vi "test Get Set EST CD.vi"(8 "error in (no error)":errorcluster, 11 "TestCase in":refnum<class "Scripting API Test Case.lvclass">) -> (0 "error out":errorcluster, 3 "TestCase out":refnum<class "Scripting API Test Case.lvclass">)   [LabVIEW 2020, in "Scripting API Test Case.lvclass"]
uses:
  Scripting API Test Case.lvclass
  Scripting API/Custom Device/Engine Simulation Toolkit Custom Device Settings.ctl
  Scripting API Test Case.lvclass/Scripting API Test Case.ctl
  <vilib>/addons/_JKI Toolkits/VI Tester/TestCase.llb/TestCase.lvclass
  Scripting API/Engine Simulation Toolkit Scripting API.lvlib
  C:/Program Files (x86)/National Instruments/LabVIEW 2020/vi.lib/addons/_JKI Toolkits/VI Tester/TestCase.llb/TestCase.lvclass
panel:
  in  "Save?":bool
  out "Output Filename":string
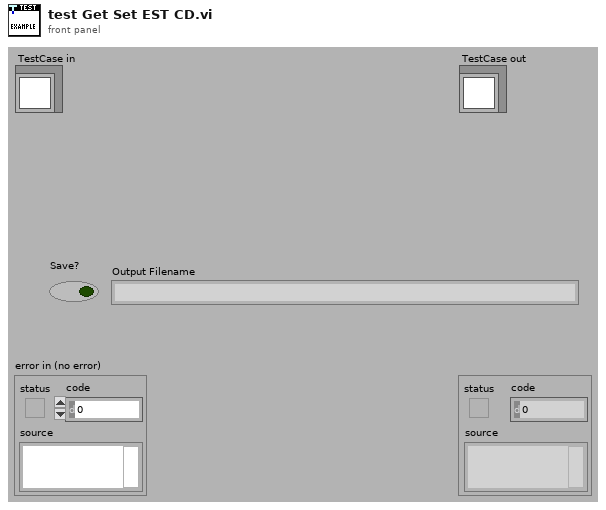
[diagram p1: front panel]
types:
  T1 = typedef "Engine Simulation Toolkit Scripting API.lvlib/Engine Simulation Toolkit Custom Device Settings.ctl" = cluster{"Name":string, "Execution priority":enum16{"Low", "Medium", "High"}, "Rate decimation":i32, "CPU":i32}
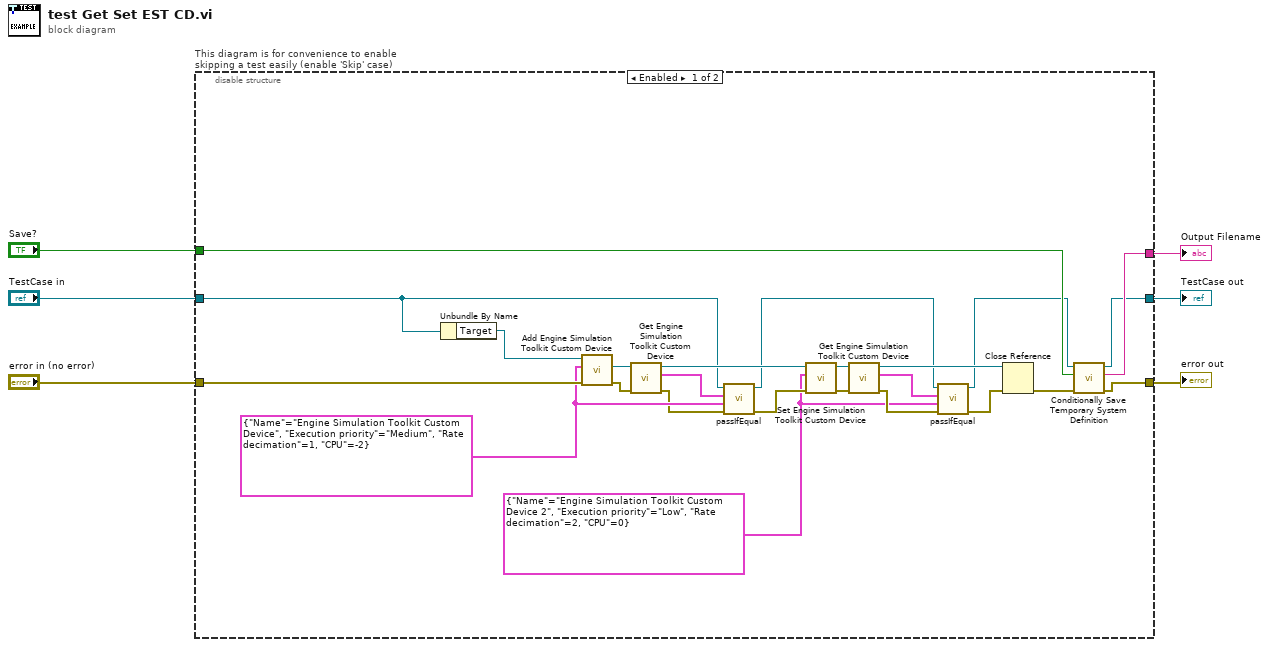
[diagram p0: block diagram]
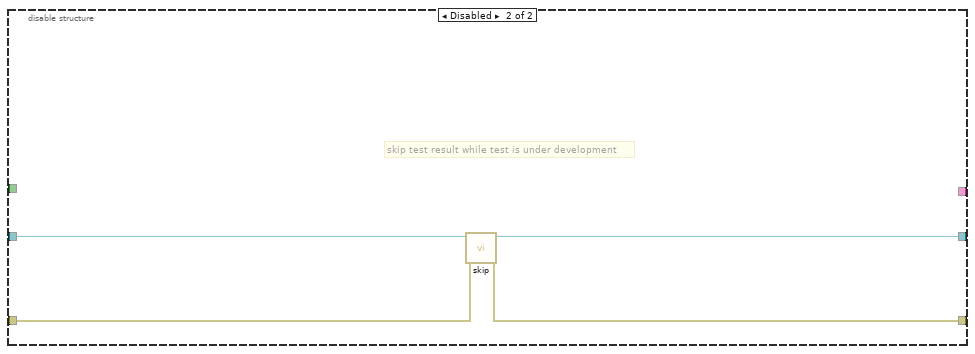
[diagram p2: hidden frame]
diagram:
  n1 = disable-structure "This diagram is for convenience to enable skipping a test easily (enable 'Skip' case)" shown="Enabled" {
    disable-tunnel: "TestCase in" -> [w10 w34]
    disable-tunnel: [w7 w32] -> w3
    disable-tunnel: [w29 w33] -> w5
    disable-tunnel: "error in (no error)" -> [w30 w31]
    disable-tunnel: [w28 _] -> w2
    disable-tunnel: "Save?" -> [w27 _]
    frame Enabled {
      w11 = T1 {"Name"="Engine Simulation Toolkit Custom Device 2", "Execution priority"=enum."Low", "Rate decimation"=2, "CPU"=0} ("Engine Simulation Toolkit Custom Device Settings")
      w20 = T1 {"Name"="Engine Simulation Toolkit Custom Device", "Execution priority"=enum."Medium", "Rate decimation"=1, "CPU"=-2} ("Engine Simulation Toolkit Custom Device Settings")
      n2 = Unbundle By Name(w10) -> ("Target"=w9:refnum<k24>)
      n3 = call "Add Engine Simulation Toolkit Custom Device.vi"("error in (no error)"=w30, "Settings"=w20, "Target in"=w9) -> ("error out"=w23:errorcluster, "EST Custom Device"=w22:refnum<k24>)  [unwired: 6 in, 1 out]
      n4 = call "Get Engine Simulation Toolkit Custom Device.vi"("error in (no error)"=w23, "EST Custom Device in"=w22) -> ("error out"=w16:errorcluster, "Settings"=w21:T1, "EST Custom Device out"=w24:refnum<k24>)  [unwired: 7 in]
      n5 = call-dynamic "passIfEqual.vi"("error in (no error)"=w16, "y"=w20, "x"=w21, "TestCase in"=w10) -> ("error out"=w17:errorcluster, "TestCase out"=w13:refnum<class "Scripting API Test Case.lvclass">)  [unwired: 6 in]
      n6 = call "Set Engine Simulation Toolkit Custom Device.vi"("error in (no error)"=w17, "Settings"=w11, "EST Custom Device in"=w24) -> ("error out"=w26:errorcluster, "EST Custom Device out"=w25:refnum<k24>)  [unwired: 7 in]
      n7 = call "Get Engine Simulation Toolkit Custom Device.vi"("error in (no error)"=w26, "EST Custom Device in"=w25) -> ("error out"=w15:errorcluster, "Settings"=w12:T1, "EST Custom Device out"=w18:refnum<k24>)  [unwired: 7 in]
      n8 = call-dynamic "passIfEqual.vi"("error in (no error)"=w15, "y"=w11, "x"=w12, "TestCase in"=w13) -> ("error out"=w14:errorcluster, "TestCase out"=w8:refnum<class "Scripting API Test Case.lvclass">)  [unwired: 6 in]
      n9 = Close Reference(reference=w18, error in (no error)=w14) -> (error out=w19:errorcluster)
      n10 = call "Conditionally Save Temporary System Definition.vi"("error in (no error)"=w19, "Save?"=w27, "Test Case"=w8) -> ("error out"=w29:errorcluster, "filename"=w28:string, "Test Case"=w7:refnum<class "Scripting API Test Case.lvclass">)  [unwired: 6 in]
    }
    frame Disabled {
      # "skip test result while test is under development"
      n11 = call <vilib>:"skip.vi"("error in (no error)"=w31, "TestCase in"=w34) -> ("error out"=w33:errorcluster, "TestCase out"=w32:refnum<class "Scripting API Test Case.lvclass">)  [unwired: 8 in]
    }
  }
  "error out" <- w5
  "TestCase out" <- w3
  "Output Filename" <- w2
